vi "Create All Message Queues.vi"(8 "error in":errorcluster) -> (0 "error out":errorcluster, 3 "Message Queues out":T1)   [LabVIEW 2021, in "Message Queue.lvlib"]
doc: "This VI creates and initializes all the message queues for your application. If your application requires more than one message queue, right-click the \"Message Queues\" constant above and select Open Type Def. Add the new Message Queue(s) to the type definition, then initialize them in this VI."
uses:
  Message Queue.lvlib
  All Message Queues.ctl
  Message Cluster.ctl
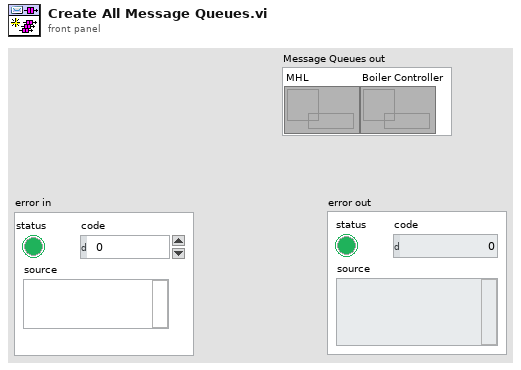
[diagram p1: front panel]
types:
  T1 = typedef "Message Queue.lvlib/All Message Queues.ctl" = cluster{"MHL":refnum<queue>, "Boiler Controller":refnum<queue>}
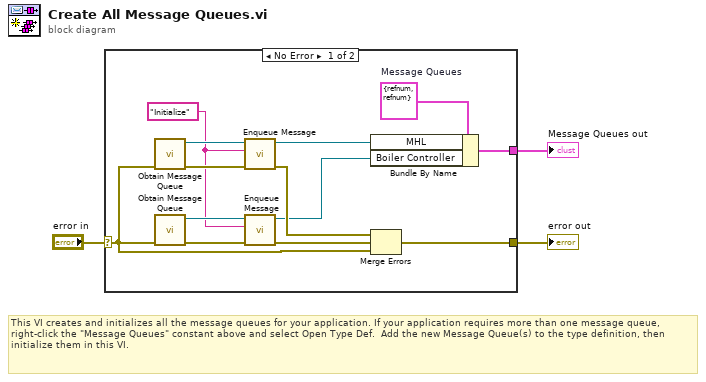
[diagram p0: block diagram]
diagram:
  # "This VI creates and initializes all the message queues for your application. If your application requires more than one message queue, right-click the \"Message Queues\" constant above and select Open Type Def.  Add the new Message Queue(s) to the type definition, then initialize them in this VI."
  n1 = case shown="No Error" "error in" {
    selector: "error in" -> [w6 w17]
    tunnel: [w9 w17] -> w2
    tunnel: [w15 _] -> w1
    frame No Error {
      w5 = "Initialize" ("Message")
      w16 = T1 {"MHL"=refnum, "Boiler Controller"=refnum}  # Message Queues
      n2 = call "Obtain Message Queue.vi"("error in"=w6) -> ("error out"=w12:errorcluster, "Message Queue"=w13:refnum<queue>)  [unwired: 9 in]
      n3 = call "Obtain Message Queue.vi"("error in"=w6) -> ("error out"=w14:errorcluster, "Message Queue"=w10:refnum<queue>)  [unwired: 9 in]
      n4 = call "Enqueue Message.vi"("error in"=w12, "Message"=w5, "Message Queue"=w13) -> ("error out"=w7:errorcluster, "dup Message Queue"=w11:refnum<queue>)  [unwired: 7 in]
      n5 = call "Enqueue Message.vi"("error in"=w14, "Message"=w5, "Message Queue"=w10) -> ("error out"=w8:errorcluster, "dup Message Queue"=w4:refnum<queue>)  [unwired: 7 in]
      n6 = Bundle By Name(cluster=w16, "MHL"=w11, "Boiler Controller"=w4) -> (w15:T1)
      n7 = Merge Errors(w7, w8, w6) -> (w9:errorcluster)
    }
    frame Error {
    }
  }
  "error out" <- w2
  "Message Queues out" <- w1
